vi "SLL DE Write DAQ Engine Parameters form INI File.vi"(8 "error in (no error)":errorcluster) -> (0 "error out":errorcluster)   [LabVIEW 2013]
uses:
  Controls/SLL DE DAQ Engine Parameters.ctl
  Controls/SLL DE List of Analog Outputs.ctl
  Controls/SLL DE List of Digital Outputs.ctl
  Controls/SLL DE List of Analog Inputs.ctl
  Controls/SLL DE List of AI Channel Type.ctl
  Controls/SLL DE DAQ Parameters LV2Global Options.ctl
  <vilib>/Utility/config.llb/NI_LVConfig.lvlib
panel:
  out "DAQ Engine":T1={"Enable Engines"={"AI Enable"=TRUE, "AO Enable"=TRUE, "DI Enable"=TRUE, "DO Enable"=TRUE}, "DAQ Control Type"={"Analog Input"=enum."Finite", "Analog Output"=enum."Finite", "Digital Input"=enum."Finite", "Digital Output"=enum."Finite"}, "DAQ Parameters"={"AI Sampling Rate (Samples/Sec)"=1000.0, "MvgAVG Window Size (# of Points)"=20, "Enable Filter"=TRUE, "Enable MvgAVG"=TRUE, "Circular Buffer Size (Sec)"=5.0, "AO Sampling Rate (Samples/Sec)"=1000.0, "Graph Update Rate (Samples/Sec)"=0.0, "File Logging Rate (Samples/Sec)"=500}, "AO Safe Values"=[], "DO Safe Values"=[], "DO Interconnected Lines"=[], "AI Channels Unit"=[], "Units Information"=[]}
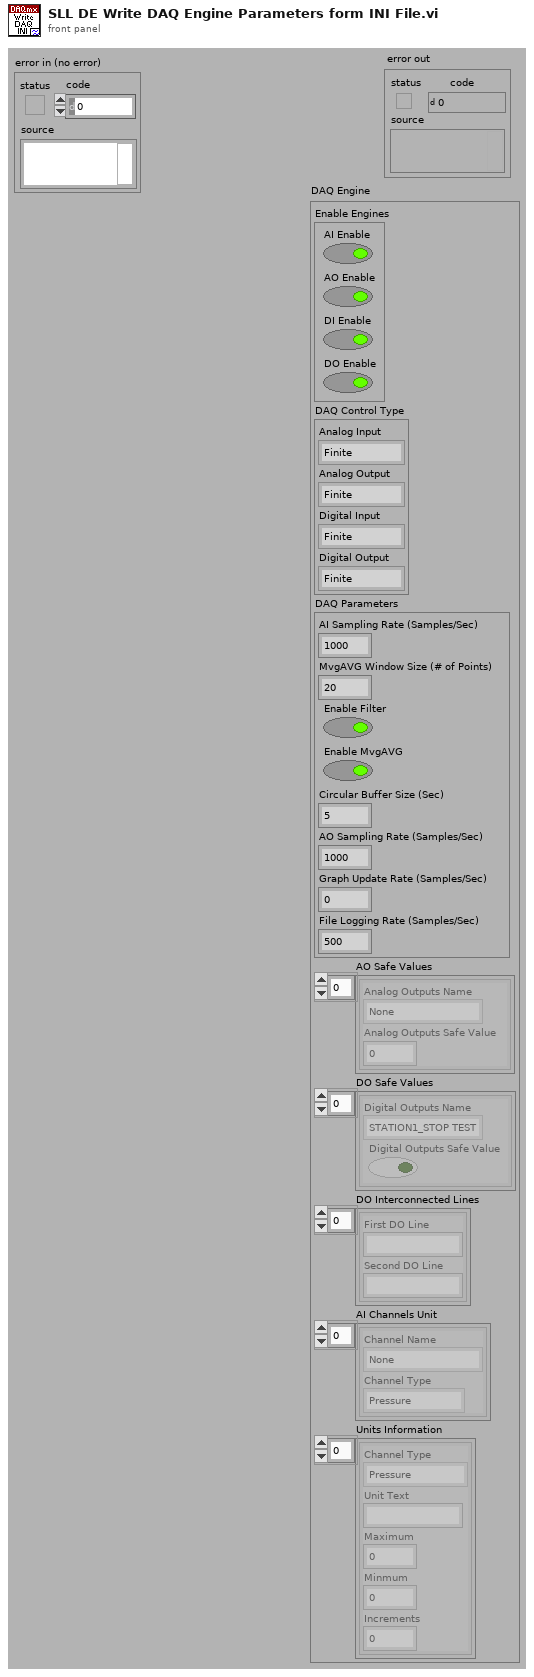
[diagram p1: front panel]
types:
  T1 = typedef "SLL DE DAQ Engine Parameters.ctl" = cluster{"Enable Engines":cluster{"AI Enable":bool, "AO Enable":bool, "DI Enable":bool, "DO Enable":bool}, "DAQ Control Type":cluster{"Analog Input":enum16{"Finite", "Continuous", "Driver"}, "Analog Output":enum16{"Finite", "Continuous", "Driver"}, "Digital Input":enum16{"Finite", "Continuous", "Driver"}, "Digital Output":enum16{"Finite", "Continuous", "Driver"}}, "DAQ Parameters":cluster{"AI Sampling Rate (Samples/Sec)":dbl, "MvgAVG Window Size (# of Points)":i32, "Enable Filter":bool, "Enable MvgAVG":bool, "Circular Buffer Size (Sec)":dbl, "AO Sampling Rate (Samples/Sec)":dbl, "Graph Update Rate (Samples/Sec)":dbl, "File Logging Rate (Samples/Sec)":i32}, "AO Safe Values":cluster{"Analog Outputs Name":T2, "Analog Outputs Safe Value":dbl}[], "DO Safe Values":cluster{"Digital Outputs Name":T3, "Digital Outputs Safe Value":bool}[], "DO Interconnected Lines":cluster{"First DO Line":string, "Second DO Line":string}[], "AI Channels Unit":cluster{"Channel Name":T4, "Channel Type":T5}[], "Units Information":cluster{"Channel Type":T5, "Unit Text":string, "Maximum":dbl, "Minmum":dbl, "Increments":dbl}[]}
  T2 = typedef "SLL DE List of Analog Outputs.ctl" = enum16{"None"}
  T3 = typedef "SLL DE List of Digital Outputs.ctl" = enum16{"STATION1_START TEST", "STATION1_STOP TEST", "STATION1_LIGHT1", "STATION1_LIGHT2", "STATION1_LIGHT3", "STATION2_START TEST", "STATION2_STOP TEST", "STATION2_LIGHT1", "STATION2_LIGHT2", "STATION2_LIGHT3", "STATION3_START TEST", "STATION3_STOP TEST", "STATION3_LIGHT1", "STATION3_LIGHT2", "STATION3_LIGHT3", "STATION4_START TEST", "STATION4_STOP TEST", "STATION4_LIGHT1", "STATION4_LIGHT2", "STATION4_LIGHT3"}
  T4 = typedef "SLL DE List of Analog Inputs.ctl" = enum16{"None"}
  T5 = typedef "SLL DE List of AI Channel Type.ctl" = enum16{"Pressure", "Flow", "Temperature", "Time Scale", "Voltage", "Current", "Frequency", "Sound", "Speed", "Torque", "Distance", "Channel Type 1", "Channel Type 2", "Channel Type 3"}
  T6 = typedef "SLL DE DAQ Parameters LV2Global Options.ctl" = enum16{"Read", "Write"}
  T7 = typedef "NI_LVConfig.lvlib/Config Data RefNum.ctl" = refnum<k1>
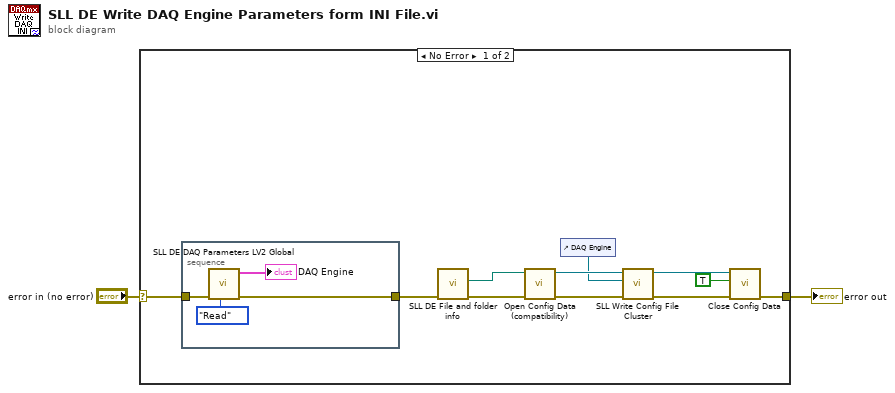
[diagram p0: block diagram]
diagram:
  n1 = case shown="No Error" "error in (no error)" {
    selector: "error in (no error)" -> [w8 w18]
    tunnel: [w10 w18] -> w1
    frame No Error {
      n2 = stacked-sequence {
        tunnel: w8 -> [w17]
        tunnel: [w16] -> w9
        frame #0 {
          n3 = call "SLL DE DAQ Parameters LV2 Global.vi"("Option"=SLL_DE_DAQ_Parameters_LV2Global_Options."Read", "Error in (no error)"=w17) -> ("Error out"=w16:errorcluster, "Global Info"=→"DAQ Engine":T1)  [unwired: 8 in]
        }
      }
      n4 = call "SLL DE File and folder info.vi"("error in (no error)"=w9) -> ("error out"=w12:errorcluster, "DAQ INI file path"=w13:path)  [unwired: 5 in, 4 out]
      n5 = call <vilib>:"Open Config Data (compatibility).vi"("error in (no error)"=w12, "configuration file path"=w13) -> ("error out"=w7:errorcluster, "refnum"=w4:T7)  [unwired: 7 in, 1 out]
      n6 = control-ref of="DAQ Engine"() -> (w3:refnum<vi>)
      n7 = call <userlib>:"SLL Write Config File Cluster.vi"("error in (no error)"=w7, "Config File Cluster Refnum in"=w3, "Config File Refnum in"=w4) -> ("error out"=w6:errorcluster, "Config File Refnum out"=w5:T7)  [unwired: 7 in]
      n8 = call <vilib>:"Close Config Data.vi"("error in (no error)"=w6, "write file if changed (T)"=TRUE ("write configuration file? (T)"), "refnum"=w5) -> ("error out"=w10:errorcluster)  [unwired: 7 in, 1 out]
    }
    frame Error {
    }
  }
  "error out" <- w1
